vi "PH_HamamatsuCamera.get Cam.vi"(0 "i ref in":refnum<vi>, 5 "error in":errorcluster) -> (14 "i ref out":refnum<vi>, 15 "Handle out":i32, 16 "Cam found":bool, 18 "Cam Error out":errorcluster, 19 "error out":errorcluster)   [LabVIEW 2014, in "PH_HamamatsuCamera.lvlib"]
doc: "This VI is trying to connect to the cam which serial number is stored at the database. This number is expected to be the 64 Bit Hexadecimal number which one can get by the help of the MAX, or to be the serial number written on the cam. In the latter case this VI is restricted to 9 cams (cam0, cam1, ... cam8) only."
uses:
  PH_HamamatsuCamera.lvlib
  PH_Basics/PH_Common/PH_Common.lvlib
  PH_Basics/PH_Cam_BaseClass/PH_Cam_BaseClass.lvlib
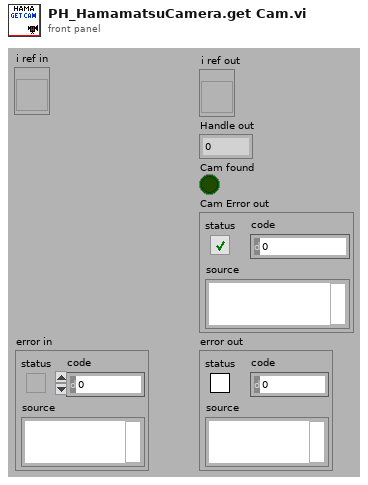
[diagram p1: front panel]
types:
  T1 = typedef "PH_Cam_BaseClass.lvlib/PH_Cam_BaseClass.i attribute.ctl" = cluster{"Gui Refs":T2, "Cam":cluster{"Source Notifier":refnum<notifier>, "Error":errorcluster, "Camera ID":string}, "Images":cluster{"Cam":T3, "Operation":T3, "PSDB":T3}, "Window Image":cluster{"Indicate Image":bool, "Window No.":i32, "Scale Facor":dbl, "Center Cross":bool, "Subtract Backgr":bool, "CoG":bool, "Color Palette":cluster{"Red":u8, "Green":u8, "Blue":u8}[], "Image On":bool}, "Default Prdc Int":i32, "Performance":cluster{"on":bool, "Timestamp Last Frame":i32}, "Histogram":cluster{"on":bool, "Mapping":bool}, "Save Image":cluster{"Save":bool, "File refnum":refnum<file>}, "Setting Service ID":i32, "Screen":cluster{"x-resolution":i16, "y-resolution":i16}, "On":bool, "Constructor finished":bool, "configured":bool}
  T2 = typedef "PH_Cam_BaseClass.lvlib/PH_Cam_BaseClass.GUI Refs.ctl" = cluster{"Frame Rate":refnum<vi>, "Get Frame Rate":refnum<vi>, "Show Image":refnum<vi>, "Get Histogram":refnum<vi>, "Mapping":refnum<vi>, "Histogram":refnum<vi>, "Center Cross":refnum<vi>, "Center of Gravity":refnum<vi>, "Scale Factor [%]":refnum<vi>, "Save Image":refnum<vi>, "Palette":refnum<vi>, "Subtract Background":refnum<vi>, "Cam Error":refnum<vi>, "On":refnum<vi>, "Cam List":refnum<vi>}
  T3 = typedef "IMAQ Image.ctl" = refnum<image>
  T4 = typedef "PH_HamamatsuCamera.lvlib/PH_HamamatsuCamera.i attribute.ctl" = cluster{"Gui Refs":cluster{"Camera Details":refnum<vi>, "ROI":refnum<vi>, "Set ROI to Maximum":refnum<vi>, "Trigger Parameters":refnum<vi>, "Brightness":refnum<vi>, "Shutter":refnum<vi>, "Gain":refnum<vi>, "Trigger Timeout":refnum<vi>, "Trigger Polarity":refnum<vi>, "Trigger Mode":refnum<vi>, "Parameters":refnum<vi>, "Set Cam Parameter":refnum<vi>, "Parameter to set":refnum<vi>, "Value to set":refnum<vi>}, "Cam":cluster{"Handle":i32, "Details":cluster{"Model":string, "Camera ID":string, "Firmware":string}, "Buffer Info":cluster{"height":u32, "width":u32, "datatype":u32}}, "H Offset":cluster{"Value":i32, "Minimum":i32, "Maximum":i32, "Increment":i32}, "V Offset":cluster{"Value":i32, "Minimum":i32, "Maximum":i32, "Increment":i32}, "H Width":cluster{"Value":i32, "Minimum":i32, "Maximum":i32, "Increment":i32}, "V Width":cluster{"Value":i32, "Minimum":i32, "Maximum":i32, "Increment":i32}, "Trigger Parameters":T5, "Trigger Timeout":u32, "Parameters":T6[], "Indicees Cam Parameters":cluster{"Brightness":i32, "Shutter":i32, "Gain":i32}, "Wanted Values":cluster{"Trigger Settings":T5[], "ROI":T7[], "Parameter":cluster{"Name":string, "Value":dbl}[]}}
  T5 = typedef "PH_HamamatsuCamera.lvlib/PH_HamamatsuCamera.Trigger Parameter.ctl" = cluster{"Mode":u32, "Polarity":u32, "Times":u32, "Delay":dbl}
  T6 = typedef "PH_HamamatsuCamera.lvlib/PH_HamamatsuCamera.Parameter Set.ctl" = cluster{"Parameter":string, "Value":dbl, "Writable":bool, "Range":cluster{"min":dbl, "max":dbl, "step":dbl}, "Default":dbl, "Value Names":cluster{"Name":string, "Value":dbl}[], "Text Values":bool}
  T7 = typedef "PH_HamamatsuCamera.lvlib/PH_HamamatsuCamera.ROI.ctl" = cluster{"Horizontal Offset":i32, "Vertical Offset":i32, "Horizontal Width":i32, "Vertical Width":i32}
  T8 = enum8{"Enabled", "Disabled", "Disabled and Grayed Out"}
  T9 = cluster{"Model":string, "Camera ID":string, "Firmware":string}
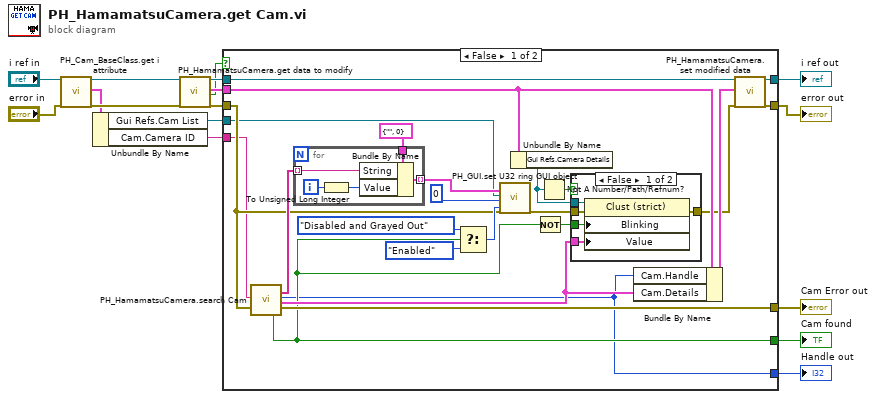
[diagram p0: block diagram]
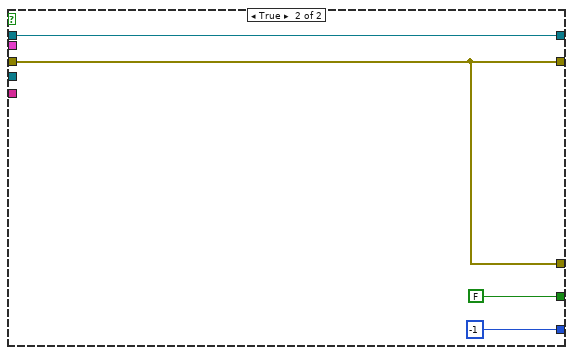
[diagram p3: hidden frame]
diagram:
  n1 = call "PH_Cam_BaseClass.get i attribute.vi"("i ref in"="i ref in", "error in (no error)"="error in") -> ("i ref out"=w5:refnum<vi>, "i attribute"=w4:T1, "error out"=w7:errorcluster)  [unwired: 15 in]
  n2 = Unbundle By Name(w4) -> ("Gui Refs.Cam List"=w2:refnum<vi>, "Cam.Camera ID"=w3:string)
  n3 = call "PH_HamamatsuCamera.get data to modify.vi"("i ref in"=w5, "error in (no error)"=w7) -> ("i ref out"=w12:refnum<vi>, "i attribute"=w11:T4, "timed out"=w9:bool, "error out"=w8:errorcluster)  [unwired: 14 in]
  n4 = case shown="False" w9 {
    tunnel: [w34 w53] -> w15
    tunnel: [w33 w55] -> w14
    tunnel: w8 -> [w24 w53]
    tunnel: [w32 w53] -> w13
    tunnel: w12 -> [w31 w55]
    tunnel: w11 -> [w30 _]
    tunnel: [w22 FALSE ("Cam found")] -> w10
    tunnel: w3 -> [w19 _]
    tunnel: w2 -> [w18 _]
    tunnel: [w17 -1 ("Handle")] -> w1
    frame False {
      n5 = call "PH_HamamatsuCamera.search Cam.vi"("Wanted Cam"=w19, "Cam Error in"=w24) -> ("Cam found"=w22:bool, "Available Cams"=w29:string[], "Handle"=w17:i32, "Camera Details"=w28:T9, "Cam Error out"=w32:errorcluster)  [unwired: 13 in]
      n6 = for {
        tunnel: cluster{"String":string, "Value":u32} {"String"="", "Value"=0} -> [w51]
        tunnel: [w50] -> w40 mode=indexing
        tunnel: w29 -> [w47] mode=indexing
        i -> [w49]
        n7 = To Unsigned Long Integer(number=w49) -> (unsigned 32bit integer=w48:u32)
        n8 = Bundle By Name(cluster=w51, "String"=w47, "Value"=w48) -> (w50:cluster{"String":string, "Value":u32})
      }
      n9 = Select(t=T8."Disabled and Grayed Out" ("Disabled"), s=w22, f=T8."Enabled" ("Disabled")) -> (s? t:f=w35:T8)
      n10 = call "PH_GUI.set U32 ring GUI object.vi"("Strings And Values [Empty]"=w40, "Ring Ref"=w18, "Value"=u32 0, "error in (no error)"=w24, "Disabled (Enabled)"=w35) -> ("error out"=w27:errorcluster)  [unwired: 14 in]
      n11 = Unbundle By Name(w30) -> ("Gui Refs.Camera Details"=w23:refnum<vi>)
      n12 = Not(x=w22) -> (.not. x?=w21:bool)
      n13 = Not A Number/Path/Refnum?(number/path/refnum=w23) -> (NaN/Path/Refnum?=w25:bool)
      n14 = case shown="False" w25 {
        tunnel: w27 -> [w45 w46]
        tunnel: [w44 w46] -> w20
        tunnel: w23 -> [w43 _]
        tunnel: w28 -> [w42 _]
        tunnel: w21 -> [w41 _]
        frame False {
          n15 = property class="Clust (strict)"(reference=w43, error in=w45, "Blinking"=w41, "Value"=w42) -> (error out=w44:errorcluster)  [unwired: 1 out]
        }
        frame True {
        }
      }
      n16 = Bundle By Name(cluster=w30, "Cam.Handle"=w17, "Cam.Details"=w28) -> (w26:T4)
      n17 = call "PH_HamamatsuCamera.set modified data.vi"("i ref in"=w31, "i attribute"=w26, "error in (no error)"=w20) -> ("i ref out"=w33:refnum<vi>, "error out"=w34:errorcluster)  [unwired: 15 in]
    }
    frame True {
    }
  }
  "Cam found" <- w10
  "i ref out" <- w14
  "error out" <- w15
  "Cam Error out" <- w13
  "Handle out" <- w1
